vi "Make_Sine.vi"(1 "N_steps_1":i32 min=0 step=1) -> (0 "SineWaveform":dbl[](array[numeric]) format="%.2f")   [LabVIEW 2013]
uses:
  <vilib>/gmath/NI_Gmath.lvlib
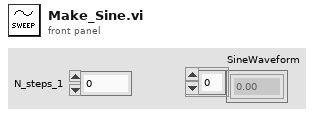
[diagram p1: front panel]
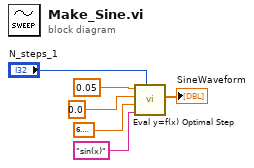
[diagram p0: block diagram]
diagram:
  n1 = call <vilib>:"Eval y=f(x) Optimal Step.vi"("number of points"="N_steps_1", "formula"="sin(x)", "end"=6.283185307179586, "start"=0.0, "epsilon"=0.05) -> ("Y Values"=→"SineWaveform":dbl[])  [unwired: 3 out]
